vi "GLOBALShooter.vi"() -> ()   [LabVIEW 2011]
panel:
  in  "Right Teleop Limit":dbl=3.55
  in  "Right Auton Limit":dbl=4.7
  out "ShooterArray":dbl[][](array[numeric]) format="%0.3f"
  out "Shooter Output":dbl
  in  "Shooter Primed":bool
  in  "Volt Prior Home":dbl
  in  "Home Position":dbl=2.5
  in  "Right Limit":dbl=3.55
  in  "Left Limit":dbl=1.45
  in  "Turret Case":dbl
  out "Turret Output":dbl
  out "Current Default Speed":dbl
  in  "Fender Default Speed":dbl=0.41
  in  "Key Default Speed":dbl=0.75
  out "Target Distance":dbl
  out "Lock On Lights":dbl
  out "Raw Turret":dbl
  # "Setpoints"
  # "Outputs/Inputs"
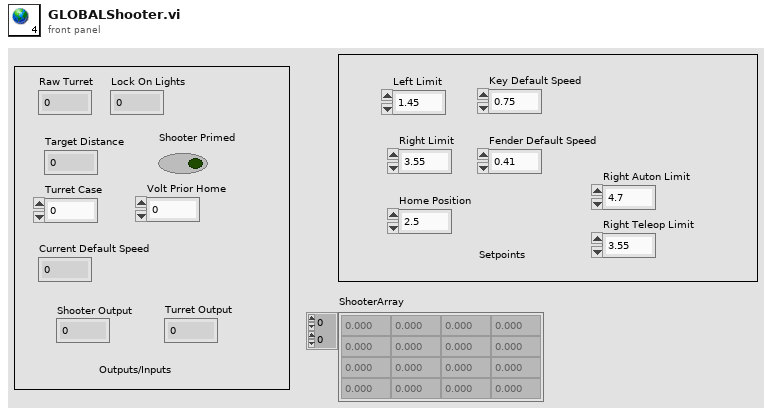
[diagram p1: front panel]
diagram:
